vi "Configure Trigger (Edge).vi"(0 "VISA resource name":refnum<visa-resource-name>, 1 "Trigger Slope (0: Positive)":u16(ring) items=["Positive", "Negative", "Alternation"], 5 "Trigger Source (0: Channel 1)":i32(ring) items=["Channel 1", "Channel 2", "Channel 3", "Channel 4", "EXT", "EXT5", "AC Line", "Digital 0", "Digital 1", "Digital 2", "Digital 3", "Digital 4", "Digital 5", "Digital 6", "Digital 7", "Digital 8", "Digital 9", "Digital 10", "Digital 11", "Digital 12", "Digital 13", "Digital 14", "Digital 15"], 7 "Trigger Level (0.0 V)":dbl, 11 "error in (no error)":errorcluster) -> (4 "VISA resource name out":refnum<visa-resource-name>, 15 "error out":errorcluster)   [LabVIEW 2012, in "RIGOL DS1000 Series.lvlib"]
doc: "Configures edge trigger settings for an oscilloscope."
uses:
  RIGOL DS1000 Series.lvlib
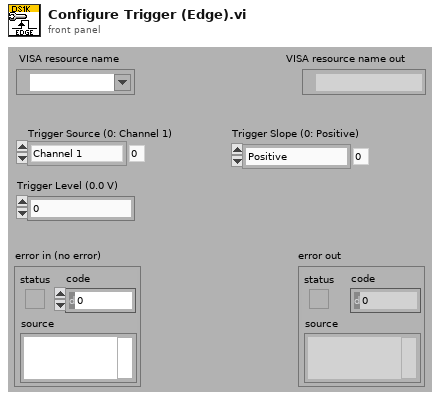
[diagram p1: front panel]
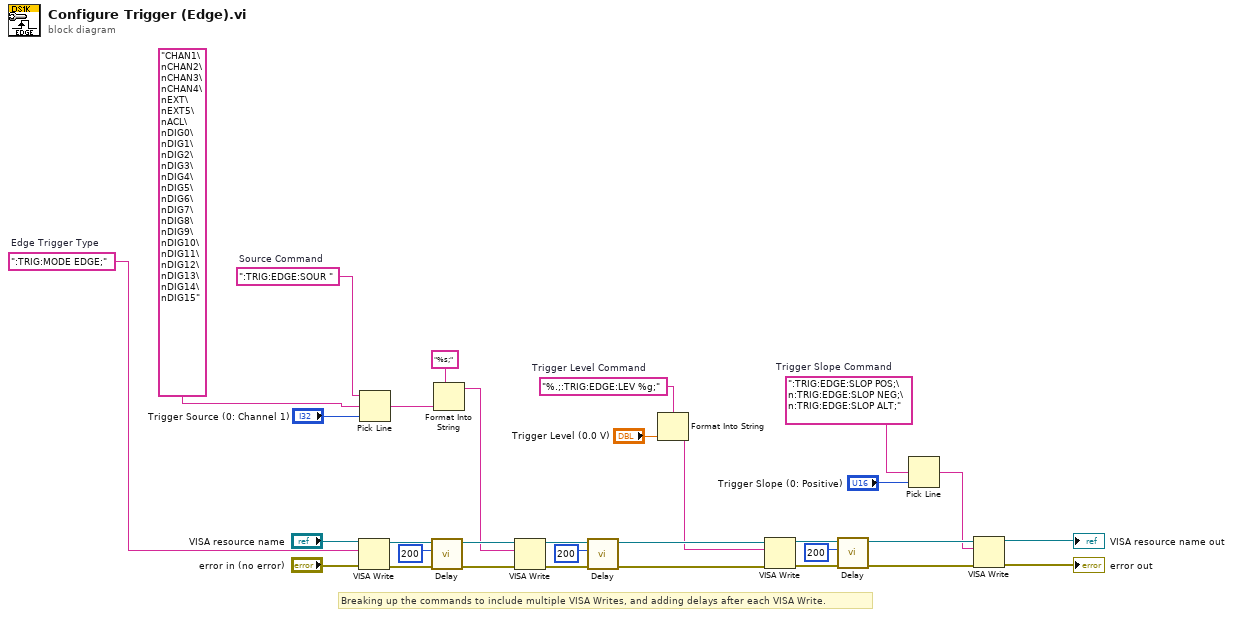
[diagram p0: block diagram]
diagram:
  w30 = ":TRIG:EDGE:SLOP POS;\n:TRIG:EDGE:SLOP NEG;\n:TRIG:EDGE:SLOP ALT;"  # Trigger Slope Command
  w32 = "%.;:TRIG:EDGE:LEV %g;"  # Trigger Level Command
  w22 = ":TRIG:MODE EDGE;"  # Edge Trigger Type
  w28 = ":TRIG:EDGE:SOUR "  # Source Command
  # "Breaking up the commands to include multiple VISA Writes, and adding delays after each VISA Write."
  n1 = VISA Write(VISA resource name="VISA resource name", write buffer=w22, error in (no error)="error in (no error)") -> (VISA resource name out=w27:refnum<visa-resource-name>, error out=w26:errorcluster)  [unwired: 1 out]
  n2 = Pick Line(string ("")=w28, multi-line string="CHAN1\nCHAN2\nCHAN3\nCHAN4\nEXT\nEXT5\nACL\nDIG0\nDIG1\nDIG2\nDIG3\nDIG4\nDIG5\nDIG6\nDIG7\nDIG8\nDIG9\nDIG10\nDIG11\nDIG12\nDIG13\nDIG14\nDIG15" ("多行字符串"), line index="Trigger Source (0: Channel 1)") -> (output string=w21:string)
  n3 = call "Delay.vi"("error in (no error)"=w26, "Delay (ms)"=u32 200, "VISA resource name"=w27) -> ("error out"=w16:errorcluster, "VISA resource name out"=w17:refnum<visa-resource-name>)  [unwired: 7 out]
  n4 = Format Into String(format string="%s;", w21) -> (resulting string=w15:string)  [unwired: 2 in, 1 out]
  n5 = VISA Write(VISA resource name=w17, write buffer=w15, error in (no error)=w16) -> (VISA resource name out=w20:refnum<visa-resource-name>, error out=w19:errorcluster)  [unwired: 1 out]
  n6 = call "Delay.vi"("error in (no error)"=w19, "Delay (ms)"=u32 200, "VISA resource name"=w20) -> ("error out"=w10:errorcluster, "VISA resource name out"=w11:refnum<visa-resource-name>)  [unwired: 7 out]
  n7 = Format Into String(format string=w32, "Trigger Level (0.0 V)") -> (resulting string=w9:string)  [unwired: 2 in, 1 out]
  n8 = VISA Write(VISA resource name=w11, write buffer=w9, error in (no error)=w10) -> (VISA resource name out=w14:refnum<visa-resource-name>, error out=w13:errorcluster)  [unwired: 1 out]
  n9 = call "Delay.vi"("error in (no error)"=w13, "Delay (ms)"=u32 200, "VISA resource name"=w14) -> ("error out"=w7:errorcluster, "VISA resource name out"=w8:refnum<visa-resource-name>)  [unwired: 7 out]
  n10 = Pick Line(multi-line string=w30, line index="Trigger Slope (0: Positive)") -> (output string=w6:string)  [unwired: 1 out]
  n11 = VISA Write(VISA resource name=w8, write buffer=w6, error in (no error)=w7) -> (VISA resource name out=→"VISA resource name out":refnum<visa-resource-name>, error out=→"error out":errorcluster)  [unwired: 1 out]
